vi "Save Map of Asked Questions to Disk.vi"(8 "error in (no error)":errorcluster, 10 "Asked Questions and Answers":cluster{"String":string, "String":string}[](array[cluster]), 11 "Asked Questions":path) -> ()   [LabVIEW 2024, in "Controller.lvlib" / "Controller.lvclass"]
uses:
  Controller.lvclass
  Controller.lvclass/Controller.ctl
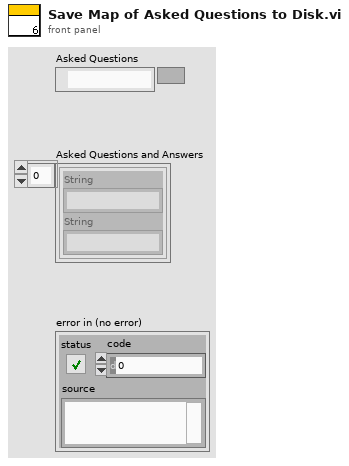
[diagram p1: front panel]
types:
  T1 = enum16{"open", "replace", "create", "open or create", "replace or create", "replace or create with confirmation"}
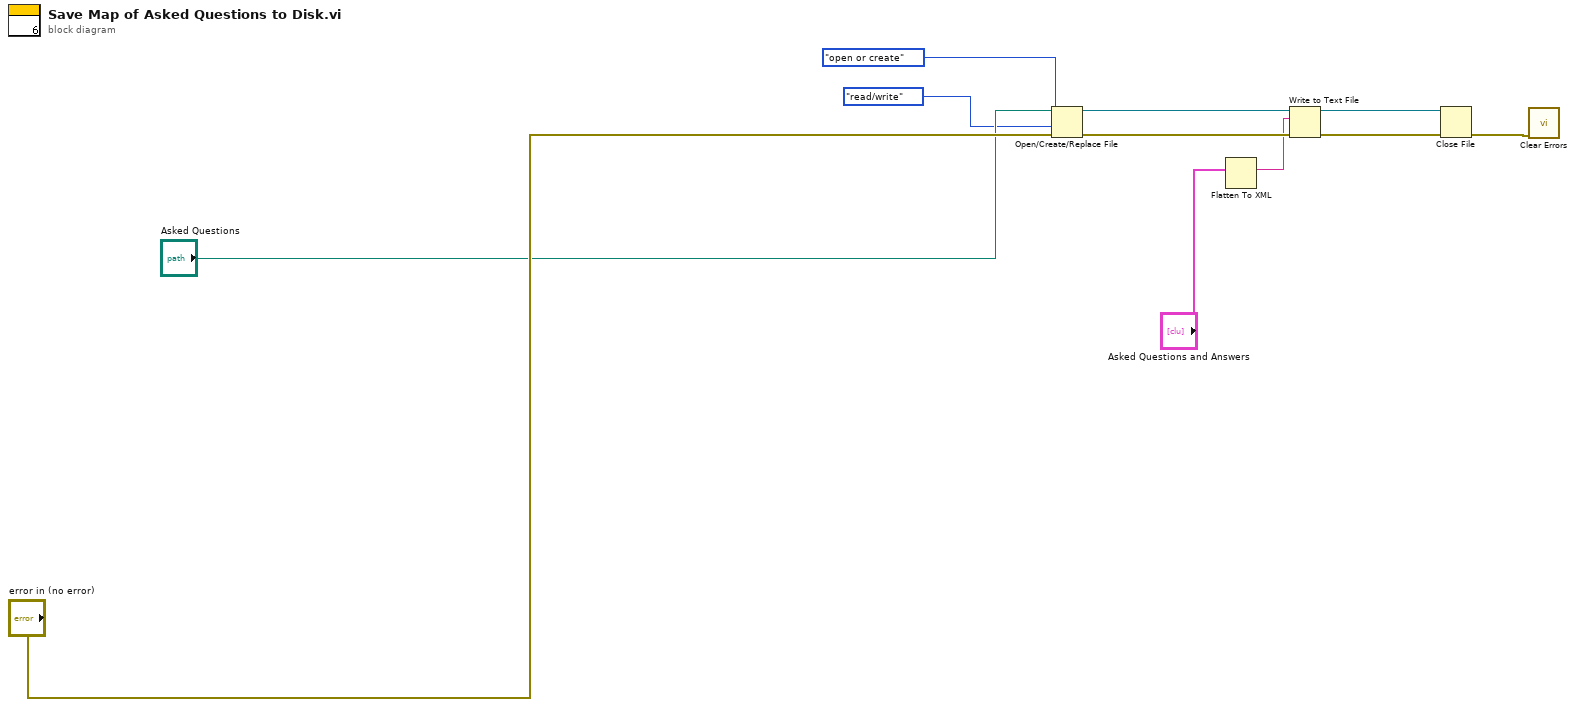
[diagram p0: block diagram]
diagram:
  n1 = Open/Create/Replace File(file path (use dialog)="Asked Questions", error in="error in (no error)", operation (0:open)=T1."open or create", access (0:read/write)=enum16{"read/write", "read-only", "write-only"}."read/write") -> (refnum out=w7:refnum<file>, error out=w8:errorcluster)  [unwired: 2 in, 1 out]
  n2 = Flatten To XML(6:"Asked Questions and Answers") -> (2:w5:string)
  n3 = Write to Text File(file (use dialog)=w7, text=w5, error in=w8) -> (refnum out=w4:refnum<file>, error out=w9:errorcluster)  [unwired: 1 in, 1 out]
  n4 = Close File(refnum=w4, error in=w9) -> (error out=w10:errorcluster)  [unwired: 1 out]
  n5 = call <vilib>:"Clear Errors.vi"("error in (no error)"=w10) -> ()  [unwired: 5 in, 2 out]
